vi "ELVIS III v1.0 Reserve IRQ.vi"(4 "Callback VI Ref":T2, 5 "Allow Overwrite? (F)":bool, 6 "myRIO FPGA Ref In":T1, 7 "Is Reserve?":bool, 8 "error in (no error)":errorcluster, 9 "IO IRQ Channels Enum":T4, 10 "IRQ Type":T3, 11 "IRQ Number":u8) -> (0 "error out":errorcluster, 2 "Succeed?":bool)   [LabVIEW 2021]
uses:
  <vilib>/myRIO/Common/Instrument Driver Framework/myRIO v1.0/IRQ/typedefs/IO IRQ Channels Enum.ctl
  <vilib>/myRIO/Common/Instrument Driver Framework/myRIO v1.0/IRQ/typedefs/IRQ Type.ctl
  <vilib>/myRIO/Common/Instrument Driver Framework/myRIO v1.0/IRQ/typedefs/Callback VI Ref.ctl
  <vilib>/myRIO/Common/Instrument Driver Framework/Utilities/typedefs/Generic FPGA Reference.ctl
  <vilib>/myRIO/Common/Instrument Driver Framework/Utilities/typedefs/FPGA Ref Manager Action Enum.ctl
  <vilib>/myRIO/Common/Instrument Driver Framework/myRIO v1.0/IRQ/typedefs/Timer IRQ FPGA Reference.ctl
  <vilib>/myRIO/Common/Instrument Driver Framework/myRIO v1.0/IRQ/typedefs/Generic IRQ.ctl
  <vilib>/myRIO/Common/Instrument Driver Framework/ELVIS III v1.0/IRQ/vis/ELVIS III v1.0 Build MUX Configuration AI IRQ.vi
  <vilib>/rvi/errors/niLvFpgaAdjustHostInterfaceError.vi
  <vilib>/myRIO/Common/Instrument Driver Framework/ELVIS III v1.0/Resource Manager/vis/ELVIS III v1.0 Unreserve Channel List.vi
  <vilib>/rvi/interface/nirviReadWriteControl/nirviReadWriteControl.xnode
  NiFpgaLv.dll
  <vilib>/rvi/interface/Simulation/niFpgaSimulationCallBeginRW.vi
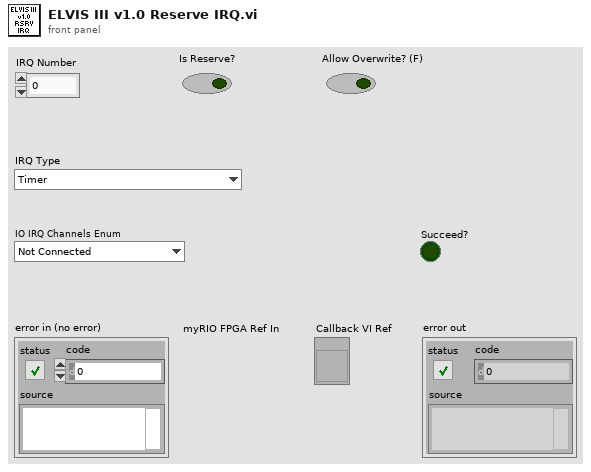
[diagram p1: front panel]
types:
  T1 = typedef "Generic FPGA Reference.ctl" = refnum<k20>
  T2 = typedef "Callback VI Ref.ctl" = refnum<vi>
  T3 = typedef "IRQ Type.ctl" = enum16{"Timer", "Analog falling edge", "Analog rising edge", "Digital falling edge", "Digital rising edge", "Digital edge"}
  T4 = typedef "IO IRQ Channels Enum.ctl" = enum16{"Not Connected", "A/AI0 (Interrupt)", "A/AI1 (Interrupt)", "A/DIO0 (Interrupt)", "A/DIO1 (Interrupt)", "A/DIO2 (Interrupt)", "A/DIO3 (Interrupt)", "Button0 (Interrupt)", "B/AI0 (Interrupt)", "B/AI1 (Interrupt)", "B/DIO0 (Interrupt)", "B/DIO1 (Interrupt)", "B/DIO2 (Interrupt)", "B/DIO3 (Interrupt)"}
  T5 = typedef "FPGA Ref Manager Action Enum.ctl" = enum16{"Get", "Set", "Reset"}
  T6 = typedef "Generic IRQ.ctl" = cluster{"IRQ Type":T3, "IO IRQ Channels Enum":T4, "Callback VI Ref":T2, "Allow Overwrite?":bool, "Interrupt enabled?":bool}
  T7 = typedef "Generic IRQ Array.ctl" = T6[]
  T8 = typedef "Timer IRQ FPGA Reference.ctl" = refnum<k20>
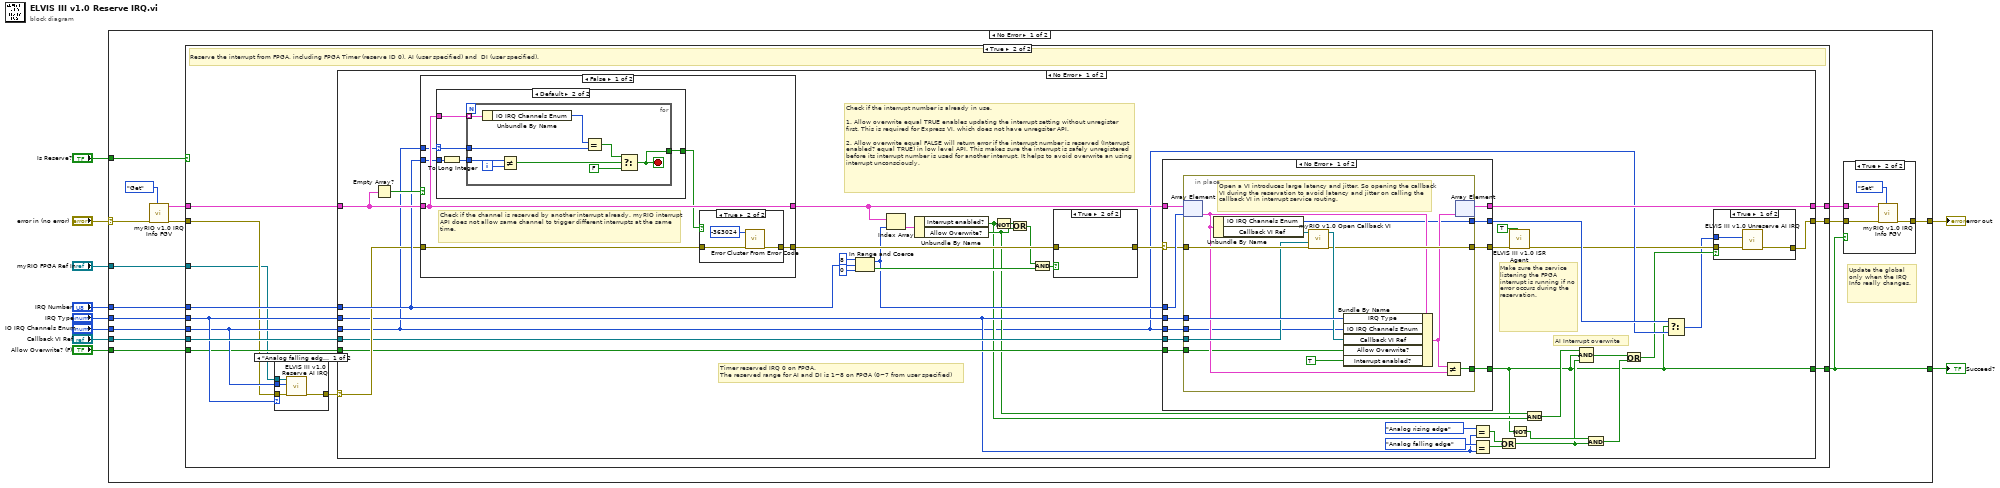
[diagram p0: block diagram]
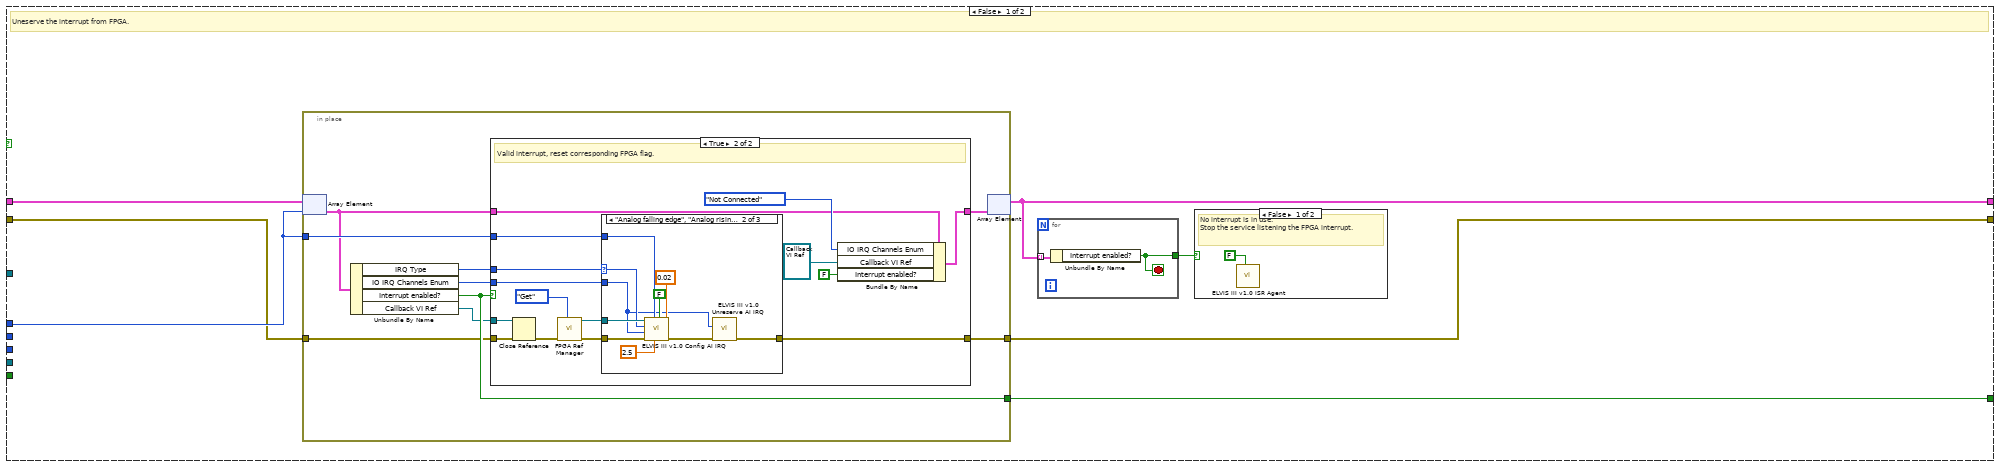
[diagram p2: hidden frame]
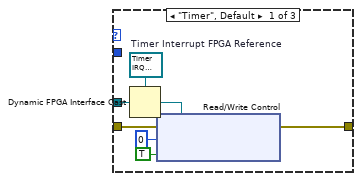
[diagram p5: hidden frame]
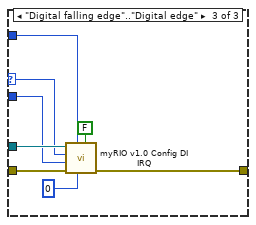
[diagram p6: hidden frame]
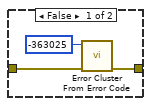
[diagram p8: hidden frame]
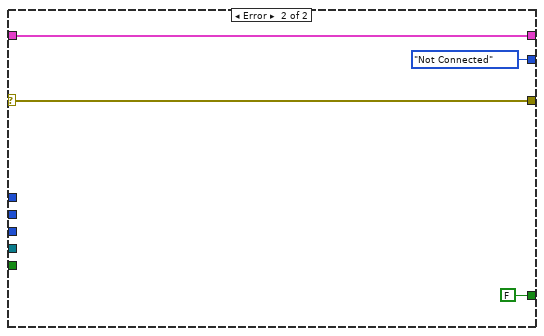
[diagram p9: hidden frame]
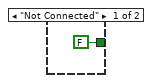
[diagram p11: hidden frame]
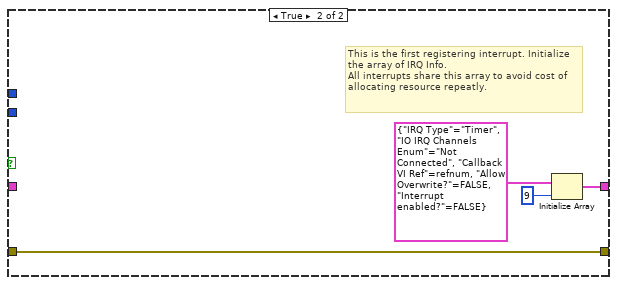
[diagram p12: hidden frame]
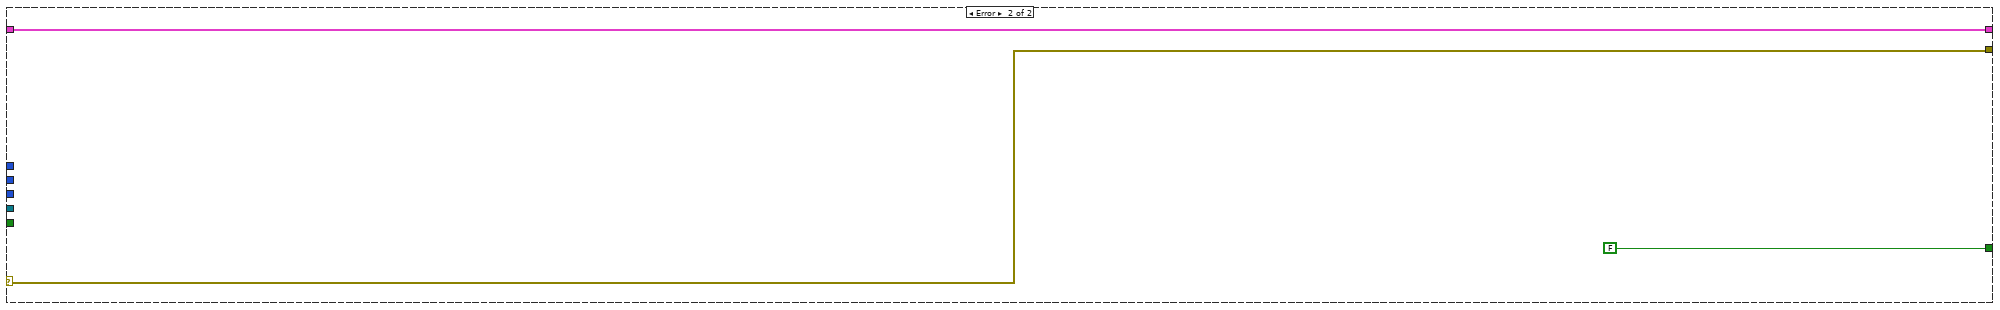
[diagram p13: hidden frame]
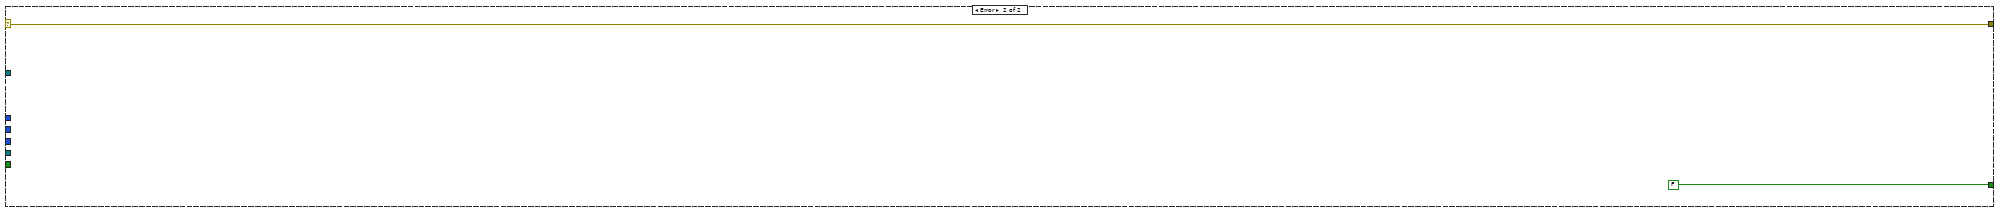
[diagram p16: hidden frame]
diagram:
  n1 = case shown="No Error" "error in (no error)" {
    selector: "error in (no error)" -> [w12 w216]
    tunnel: "IRQ Type" -> [w25 _]
    tunnel: "Callback VI Ref" -> [w24 _]
    tunnel: "Allow Overwrite? (F)" -> [w23 _]
    tunnel: [w22 w216] -> w7
    tunnel: "IO IRQ Channels Enum" -> [w21 _]
    tunnel: "IRQ Number" -> [w18 _]
    tunnel: [w15 FALSE ("Interrupt enabled?")] -> w4
    tunnel: "Is Reserve?" -> [w13 _]
    tunnel: "myRIO FPGA Ref In" -> [w11 _]
    frame No Error {
      # "Update the global only when the IRQ Info really changes."
      n2 = call <vilib>:"myRIO v1.0 IRQ Info FGV.vi"("Action"=FPGA_Ref_Manager_Action_Enum."Get", "error in (no error)"=w12) -> ("error out"=w14:errorcluster, "Generic IRQ Info out"=w20:T7)  [unwired: 8 in]
      n3 = case shown="True" w13 {
        tunnel: w25 -> [_ w92]
        tunnel: w24 -> [_ w98]
        tunnel: w23 -> [_ w90]
        tunnel: w21 -> [_ w91]
        tunnel: w20 -> [w30 w97]
        tunnel: w18 -> [w31 w96]
        tunnel: [w28 w95] -> w17
        tunnel: [w26 w93] -> w16
        tunnel: [w27 w94] -> w15
        tunnel: w14 -> [w29 w89]
        tunnel: w11 -> [_ w87]
        frame False {
          # "Uneserve the interrupt from FPGA."
          n4 = in-place {
            in-place-border: [w43] -> w27
            in-place-border: w31 -> [w41]
            in-place-border: w29 -> [w39]
            in-place-border: [w38] -> w26
            n5 = in-place-array #1(w30, w31) -> (w36:T6)
            n6 = Unbundle By Name(w36) -> ("IRQ Type"=w42:T3, "IO IRQ Channels Enum"=w40:T4, "Interrupt enabled?"=w43:bool, "Callback VI Ref"=w37:T2)
            n7 = case shown="True" w43 {
              tunnel: [w46 w61] -> w44
              tunnel: w36 -> [w46 w57]
              tunnel: w42 -> [_ w56]
              tunnel: w41 -> [_ w53]
              tunnel: w40 -> [_ w52]
              tunnel: w39 -> [w45 w49]
              tunnel: [w45 w50] -> w38
              tunnel: w37 -> [_ w47]
              frame False {
                # "Invalid interrupt, do nothing."
              }
              frame True {
                # "Valid interrupt, reset corresponding FPGA flag."
                n8 = Close Reference(reference=w47, error in (no error)=w49) -> (error out=w48:errorcluster)
                n9 = call <vilib>:"FPGA Ref Manager.vi"("Action"=FPGA_Ref_Manager_Action_Enum."Get", "error in (no error)"=w48) -> ("error out"=w51:errorcluster, "Generic FPGA Reference out"=w54:T1)  [unwired: 7 in]
                n10 = case shown="\"Analog falling edge\", \"Analog rising edge\"" w56 {
                  selector: w56 -> [_ w75 w83]
                  tunnel: w54 -> [w65 w78 w84]
                  tunnel: w53 -> [_ w77 w85]
                  tunnel: w52 -> [_ w71 w82]
                  tunnel: w51 -> [w64 w74 w81]
                  tunnel: [w63 w69 w79] -> w50
                  frame "Timer", Default {
                    w62 = T8 refnum  # Timer Interrupt FPGA Reference
                    n11 = Dynamic FPGA Interface Cast(Session In=w62, Type=w65) -> (Session Out=w68:T8)
                    n12 = xnode "Read/Write Control"("FPGA VI Reference In"=w68, "error in"=w64, "IRQ.TIMER.WRITE"=u32 0 ("Timeout"), "IRQ.TIMER.SETTIME"=TRUE ("TIMER.SetTime")) -> ("error out"=w63:errorcluster)  [unwired: 1 out]
                  }
                  frame "Analog falling edge", "Analog rising edge" {
                    n13 = call <vilib>:"ELVIS III v1.0 Config AI IRQ.vi"("Hysteresis"=0.02, "Enable IRQ?"=FALSE, "Threshold"=2.5, "IRQ Number"=w77, "error in (no error)"=w74, "IO IRQ Channels Enum"=w71, "IRQ Type"=w75, "myRIO FPGA Ref In"=w78) -> ("error out"=w70:errorcluster)  [unwired: 3 in]
                    n14 = call <vilib>:"ELVIS III v1.0 Unreserve AI IRQ.vi"("error in (no error)"=w70, "IO IRQ Channels Enum"=w71) -> ("error out"=w69:errorcluster)  [unwired: 9 in]
                  }
                  frame "Digital falling edge".."Digital edge" {
                    n15 = call <vilib>:"myRIO v1.0 Config DI IRQ.vi"("Enable IRQ?"=FALSE, "Edge Count"=u32 0, "IRQ Number"=w85, "error in (no error)"=w81, "IO IRQ Channels Enum"=w82, "IRQ Type"=w83, "myRIO FPGA Ref In"=w84) -> ("error out"=w79:errorcluster)  [unwired: 4 in]
                  }
                }
                n16 = Bundle By Name(cluster=w57, "IO IRQ Channels Enum"=IO_IRQ_Channels_Enum."Not Connected", "Callback VI Ref"=T2 refnum, "Interrupt enabled?"=FALSE) -> (w61:T6)
              }
            }
            n17 = in-place-array #1(w44) -> (w28:T7)  [unwired: 1 out]
          }
          n18 = for {
            tunnel: w28 -> [w35] mode=indexing
            tunnel: [w34] -> w32
            stop <- w34 stop-if-true
            n19 = Unbundle By Name(w35) -> ("Interrupt enabled?"=w34:bool)
          }
          n20 = case shown="False" w32 {
            frame False {
              # "No interrupt is in use.\nStop the service listening the FPGA interrupt."
              n21 = call <vilib>:"ELVIS III v1.0 ISR Agent.vi"("Run?"=FALSE) -> ()  [unwired: 10 in, 1 out]
            }
            frame True {
              # "There is interrupt still in use. Do nothing."
            }
          }
        }
        frame True {
          # "Reserve the interrupt from FPGA, including FPGA Timer (reserve ID 0), AI (user specified) and  DI (user specified)."
          n22 = case shown="\"Analog falling edge\", \"Analog rising edge\"" w92 {
            tunnel: w91 -> [w209 _]
            tunnel: w89 -> [w208 w210]
            tunnel: [w207 w210] -> w88
            tunnel: w87 -> [w206 _]
            frame "Analog falling edge", "Analog rising edge" {
              n23 = call <vilib>:"ELVIS III v1.0 Reserve AI IRQ.vi"("error in (no error)"=w208, "IO IRQ Channels Enum"=w209, "myRIO FPGA Ref In"=w206) -> ("error out"=w207:errorcluster)  [unwired: 8 in]
            }
            frame Default {
            }
          }
          n24 = case shown="No Error" w88 {
            selector: w88 -> [w120 w205]
            tunnel: w98 -> [w118 _]
            tunnel: w97 -> [w136 w204]
            tunnel: w96 -> [w124 _]
            tunnel: [w123 w204] -> w95
            tunnel: [w99 FALSE] -> w94
            tunnel: [w119 w205] -> w93
            tunnel: w92 -> [w115 _]
            tunnel: w91 -> [w105 _]
            tunnel: w90 -> [w117 _]
            frame No Error {
              # "AI Interrupt overwrite"
              # "Make sure the service listening the FPGA interrupt is running if no error occurs during the reservation."
              # "Check if the interrupt number is already in use.\n\n1. Allow overwrite equal TRUE enables updating the interrupt setting without unregister\nfirst. This is required for Express VI, which does not have unregsiter API.\n\n2. Allow overwrite equal FALSE will return error if the interrupt number is reserved (Interrupt enabled? equal TRUE) in low level API. This makes sure the interrupt is safely unregistered before its interrupt number is used for another interrupt. It helps to avoid overwrite an using interrupt unconsciously."
              # "Timer reserved IRQ 0 on FPGA. \nThe reserved range for AI and DI is 1~8 on FPGA (0~7 from user specified)"
              n25 = Empty Array?(array=w136) -> (empty?=w137:bool)
              n26 = case shown="False" w137 {
                tunnel: [w179 w200] -> w130
                tunnel: w136 -> [w179 _]
                tunnel: [w176 w199] -> w131
                tunnel: w105 -> [w178 _]
                tunnel: w124 -> [w175 _]
                tunnel: w120 -> [w174 w199]
                frame False {
                  # "Check if the channel is reserved by another interrupt already. myRIO interrupt API does not allow same channel to trigger different interrupts at the same time."
                  n27 = case shown="Default" w178 {
                    selector: w178 -> [_ w189]
                    tunnel: w179 -> [_ w185]
                    tunnel: [FALSE w188] -> w177
                    tunnel: w175 -> [_ w187]
                    frame "Not Connected" {
                    }
                    frame Default {
                      n28 = To Long Integer(number=w187) -> (32bit integer=w186:i32)
                      n29 = for {
                        tunnel: w189 -> [w197]
                        tunnel: [w191] -> w188
                        tunnel: w186 -> [w195]
                        tunnel: w185 -> [w190] mode=indexing
                        i -> [w196]
                        stop <- w191 stop-if-true
                        n30 = Unbundle By Name(w190) -> ("IO IRQ Channels Enum"=w198:T4)
                        n31 = Not Equal?(x=w195, y=w196) -> (x != y?=w194:bool)
                        n32 = Equal?(x=w198, y=w197) -> (x = y?=w192:bool)
                        n33 = Select(t=w192, s=w194, f=FALSE) -> (s? t:f=w191:bool)
                      }
                    }
                  }
                  n34 = case shown="True" w177 {
                    tunnel: [w180 w182] -> w176
                    tunnel: w174 -> [w180 w181]
                    frame False {
                    }
                    frame True {
                      n35 = call <vilib>:"Error Cluster From Error Code.vi"("error in (no error)"=w181, "error code (0)"=-363024) -> ("error out"=w182:errorcluster)  [unwired: 7 in]
                    }
                  }
                }
                frame True {
                  # "This is the first registering interrupt. Initialize the array of IRQ Info. \nAll interrupts share this array to avoid cost of allocating resource repeatly."
                  n36 = Initialize Array(T6 {"IRQ Type"=enum."Timer", "IO IRQ Channels Enum"=enum."Not Connected", "Callback VI Ref"=refnum, "Allow Overwrite?"=FALSE, "Interrupt enabled?"=FALSE} ("Interrupt Info"), 9 ("dimension size")) -> (w200:T6[])
                }
              }
              n37 = In Range and Coerce(upper limit=u8 8, x=w124, lower limit=u8 0) -> (coerced(x)=w125:u8, In Range?=w127:bool)
              n38 = Index Array(array=w130, index=w125) -> (element=w132:T6)
              n39 = Unbundle By Name(w132) -> ("Interrupt enabled?"=w109:bool, "Allow Overwrite?"=w110:bool)
              n40 = Not(x=w109) -> (.not. x?=w133:bool)
              n41 = Or(x=w133, y=w110) -> (x .or. y?=w128:bool)
              n42 = And(x=w128, y=w127) -> (x .and. y?=w126:bool)
              n43 = case shown="True" w126 {
                tunnel: [w143 w145] -> w129
                tunnel: w131 -> [w142 w145]
                frame False {
                  n44 = call <vilib>:"Error Cluster From Error Code.vi"("error in (no error)"=w142, "error code (0)"=-363025) -> ("error out"=w143:errorcluster)  [unwired: 7 in]
                }
                frame True {
                }
              }
              n45 = case shown="No Error" w129 {
                selector: w129 -> [w149 w172]
                tunnel: w105 -> [w156 _]
                tunnel: w115 -> [w155 _]
                tunnel: w118 -> [w154 _]
                tunnel: [w153 w173] -> w123
                tunnel: w130 -> [w152 w173]
                tunnel: w117 -> [w151 _]
                tunnel: w125 -> [w150 _]
                tunnel: [w148 w172] -> w121
                tunnel: [w147 FALSE] -> w99
                tunnel: [w146 IO_IRQ_Channels_Enum."Not Connected" ("IO IRQ Channels Enum")] -> w106
                frame No Error {
                  n46 = in-place {
                    in-place-border: w154 -> [w163]
                    in-place-border: w155 -> [w169]
                    in-place-border: w156 -> [w159]
                    in-place-border: w151 -> [w158]
                    in-place-border: w149 -> [w166]
                    in-place-border: [w165] -> w148
                    in-place-border: [w160] -> w147
                    in-place-border: [w157] -> w146
                    # "Open a VI introduces large latency and jitter. So opening the callback VI during the reservation to avoid latency and jitter on calling the callback VI in interrupt service routing."
                    n47 = in-place-array #2(w152, w150) -> (w161:T6)
                    n48 = Unbundle By Name(w161) -> ("IO IRQ Channels Enum"=w157:T4, "Callback VI Ref"=w164:T2)
                    n49 = call <vilib>:"myRIO v1.0 Open Callback VI.vi"("error in (no error)"=w166, "Static Ref in"=w163, "Opened VI Ref in"=w164) -> ("error out"=w165:errorcluster, "Opened VI Ref out"=w167:T2)  [unwired: 7 in]
                    n50 = Bundle By Name(cluster=w161, "IRQ Type"=w169, "IO IRQ Channels Enum"=w159, "Callback VI Ref"=w167, "Allow Overwrite?"=w158, "Interrupt enabled?"=TRUE) -> (w162:T6)
                    n51 = Not Equal?(x=w162, y=w161) -> (x != y?=w160:bool)
                    n52 = in-place-array #2(w162) -> (w153:T7)  [unwired: 1 out]
                  }
                }
                frame Error {
                }
              }
              n53 = Equal?(x=IRQ_Type."Analog rising edge", y=w115) -> (x = y?=w113:bool)
              n54 = Equal?(x=IRQ_Type."Analog falling edge", y=w115) -> (x = y?=w112:bool)
              n55 = Or(x=w113, y=w112) -> (x .or. y?=w107:bool)
              n56 = call <vilib>:"ELVIS III v1.0 ISR Agent.vi"("Run?"=TRUE, "error in (no error)"=w121) -> ("error out"=w101:errorcluster)  [unwired: 9 in]
              n57 = Not(x=w99) -> (.not. x?=w111:bool)
              n58 = And(x=w110, y=w109) -> (x .and. y?=w108:bool)
              n59 = Compound Arithmetic op=AND(w108, w99, w107) -> (w103:bool)
              n60 = And(x=w111, y=w107) -> (x .and. y?=w104:bool)
              n61 = Or(x=w103, y=w104) -> (x .or. y?=w102:bool)
              n62 = Select(t=w106, s=w99, f=w105) -> (s? t:f=w100:T4)
              n63 = case shown="True" w102 {
                tunnel: w101 -> [w140 w141]
                tunnel: [w139 w141] -> w119
                tunnel: w100 -> [w138 _]
                frame True {
                  n64 = call <vilib>:"ELVIS III v1.0 Unreserve AI IRQ.vi"("error in (no error)"=w140, "IO IRQ Channels Enum"=w138) -> ("error out"=w139:errorcluster)  [unwired: 9 in]
                }
                frame False {
                }
              }
            }
            frame Error {
            }
          }
        }
      }
      n65 = case shown="True" w15 {
        tunnel: [w211 w215] -> w22
        tunnel: w17 -> [_ w213]
        tunnel: w16 -> [w211 w212]
        frame False {
        }
        frame True {
          n66 = call <vilib>:"myRIO v1.0 IRQ Info FGV.vi"("Action"=FPGA_Ref_Manager_Action_Enum."Set", "error in (no error)"=w212, "Generic IRQ Info in"=w213) -> ("error out"=w215:errorcluster)  [unwired: 7 in, 1 out]
        }
      }
    }
    frame Error {
    }
  }
  "error out" <- w7
  "Succeed?" <- w4
